vi "loadSettings.vi"(8 "error in (no error)":errorcluster, 11 "CameraSettingsManager in":refnum<class "CameraSettingsManager.lvclass">) -> (0 "error out":errorcluster, 3 "CameraSettingsManager out":refnum<class "CameraSettingsManager.lvclass">)   [LabVIEW 2011, in "Tools.lvlib" / "Settings.lvlib" / "CameraSettingsManager.lvclass"]
uses:
  CameraSettingsManager.lvclass
  CameraSettingsManager.lvclass/CameraSettingsManager.ctl
  CameraSettingsEventsManager/cameraSettingsEventManager.lvclass
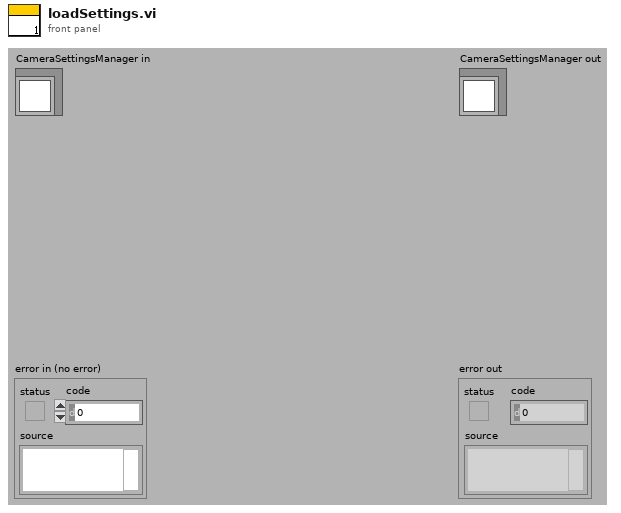
[diagram p1: front panel]
types:
  T1 = cluster{"loadCameraSettingsEvent":refnum<user-event>}
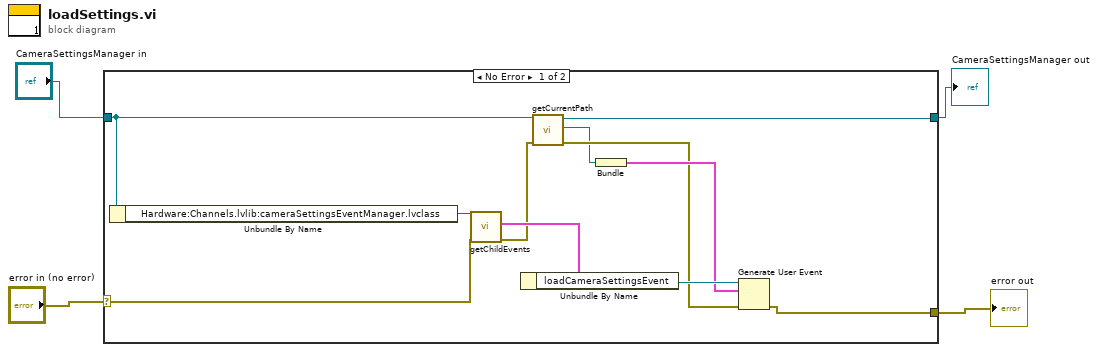
[diagram p0: block diagram]
diagram:
  n1 = case shown="No Error" "error in (no error)" {
    selector: "error in (no error)" -> [w14 w16]
    tunnel: "CameraSettingsManager in" -> [w9 w17]
    tunnel: [w5 w17] -> w3
    tunnel: [w10 w16] -> w1
    frame No Error {
      n2 = Unbundle By Name(w9) -> ("Hardware:Channels.lvlib:cameraSettingsEventManager.lvclass"=w15:refnum<class "cameraSettingsEventManager.lvclass">)
      n3 = call-dynamic "getChildEvents.vi"("error in (no error)"=w14, "cameraSettingsEventManager in"=w15) -> ("error out"=w8:errorcluster, "cameraSettingsEventsRef"=w13:T1)  [unwired: 7 in, 1 out]
      n4 = Unbundle By Name(w13) -> ("loadCameraSettingsEvent"=w12:refnum<user-event>)
      n5 = call-dynamic "getCurrentPath.vi"("error in (no error)"=w8, "SettingsManager.lvclass in"=w9) -> ("error out"=w7:errorcluster, "Current Path"=w6:path, "SettingsManager.lvclass out"=w5:refnum<class "CameraSettingsManager.lvclass">)  [unwired: 7 in]
      n6 = Bundle("Current Path"=w6) -> (w11:cluster{"Current Path":path})  [unwired: 1 in]
      n7 = Generate User Event(user event=w12, event data cluster=w11, error in=w7) -> (error out=w10:errorcluster)  [unwired: 1 out]
    }
    frame Error {
    }
  }
  "error out" <- w1
  "CameraSettingsManager out" <- w3
